vi "XLP80.vi"() -> ()   [LabVIEW 2021]
uses:
  XLP80_General_Libs/WL_Libs_V14.25/WL_TypeDefs_V14.00.llb/WL_TypeDefs_EnumState.ctl
  XLP80_General_Libs/Kirschenhofer_Libs/KH EthernetIPConfig 17.14/KH EthernetIPConfig TDef Config.ctl
  XLP80_General_Libs/Kirschenhofer_Libs/KH EthernetIPConfig 17.14/KH EthernetIPConfig TypeDefs ModuleTyp.ctl
  XLP80_ProjectLibs/XLP80_Globals/XLP80_Globals_SettingsFix.vi
  XLP80_ProjectLibs/XLP80_Globals/XLP80_Globals_Status.vi
  XLP80_General_Libs/WL_Libs_V14.25/WL_Frontpanel_V14.01.llb/WL_Frontpanel_GblStatus.vi
  XLP80_General_Libs/WL_Libs_V14.25/WL_Applications_V14.02.llb/WL_Applications_Globals.vi
  XLP80_General_Libs/Kirschenhofer_Libs/KH EthernetIP 17.19/KH_EthernetIP_Globals.vi
panel:
  out "SW-Version":string
  out "StatusLine":T1={"Status"=1, "code"=0, "source"=""}
  in  "Auto":bool
  in  "EditConf":bool
  in  "Manual":bool
  in  "Info":bool
  in  "Exit":bool
  in  "LoadConf":bool
  # "XLP 80"
  # "XLP 80"
  # "Mess- & Prüfsoftware: m-a-r-s Ing.Büro Wais; www.m-a-r-s.de"
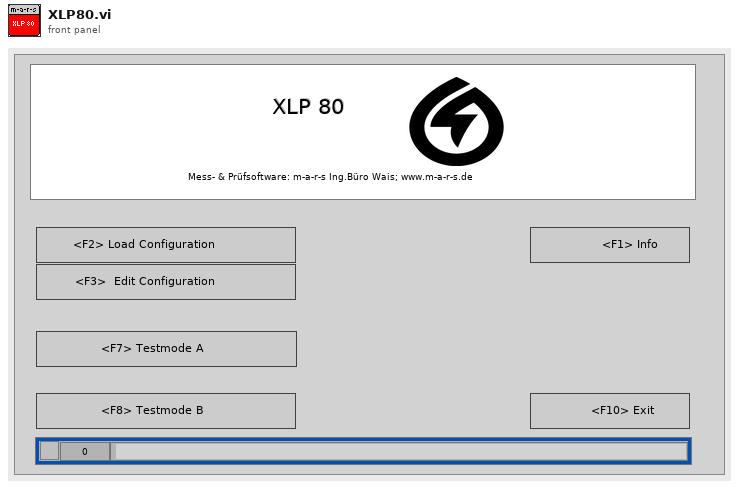
[diagram p1: front panel]
types:
  T1 = cluster{"Status":u16, "code":i32, "source":string}
  T2 = enum32{"General Settings", "Datalog", "Parameter", "AlarmReal", "AlarmBool", "AI", "AO", "DI", "DO", "CAN", "Extra Settings"}
  T3 = typedef "WL_TypeDefs_EnumState.ctl" = enum16{"Init", "Run", "End"}
  T4 = enum16{"-none-", "Info", "LoadConf", "EditConf", "Auto", "Manual", "Exit"}
  T5 = typedef "KH EthernetIPConfig TDef Config.ctl" = cluster{"Typ":T6, "Name":string, "Nr.":i32, "InputOutput":enum16{"Input", "Output"}[]}
  T6 = typedef "KH EthernetIPConfig TypeDefs ModuleTyp.ctl" = enum16{"TBEN-S2-4AI", "TBEN-S1-8DXP", "TBEN-S2-2RFID-4DXP", "TBEN-S2-4AO", "TBEN-S2-4IOL"}
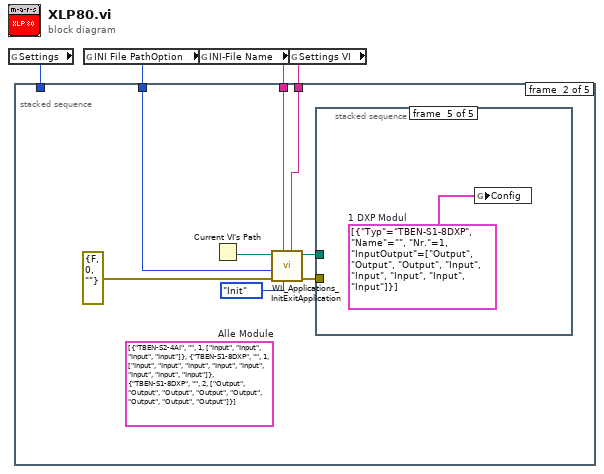
[diagram p0: block diagram]
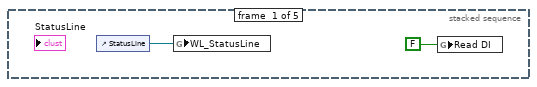
[diagram p2: hidden frame]
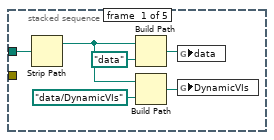
[diagram p3: hidden frame]
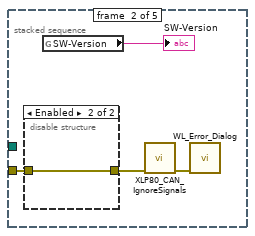
[diagram p4: hidden frame]
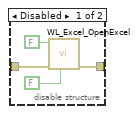
[diagram p5: hidden frame]
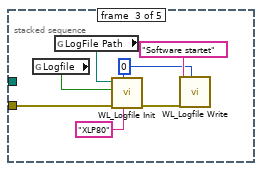
[diagram p6: hidden frame]
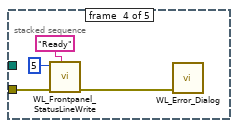
[diagram p7: hidden frame]
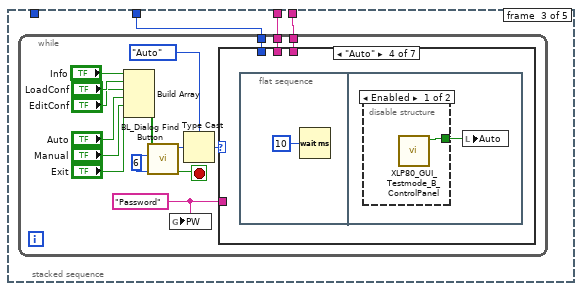
[diagram p8: hidden frame]
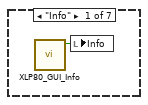
[diagram p9: hidden frame]
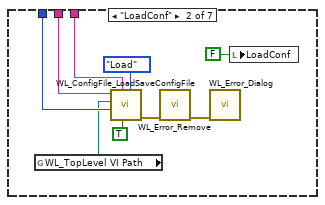
[diagram p10: hidden frame]
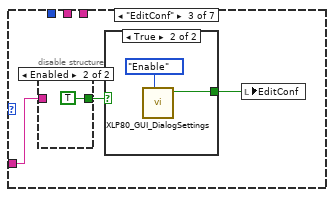
[diagram p11: hidden frame]
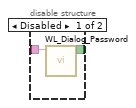
[diagram p12: hidden frame]
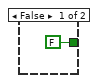
[diagram p13: hidden frame]
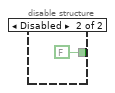
[diagram p14: hidden frame]
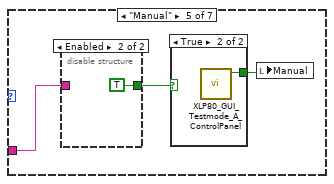
[diagram p15: hidden frame]
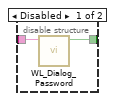
[diagram p16: hidden frame]
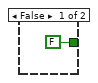
[diagram p17: hidden frame]
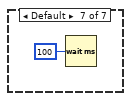
[diagram p19: hidden frame]
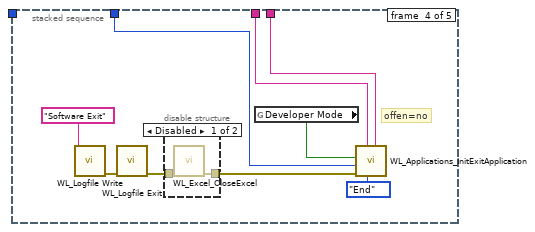
[diagram p20: hidden frame]
diagram:
  n1 = global read "Globals_Settings_XLP80.vi" "Settings"() -> (w1:T2)
  n2 = global read "XLP80_Globals_SettingsFix.vi" "INI File PathOption"() -> (w4:enum16{"WindowsPath", "LocalPath", "Path"})
  n3 = global read "XLP80_Globals_SettingsFix.vi" "INI-File Name"() -> (w3:string)
  n4 = global read "XLP80_Globals_SettingsFix.vi" "Settings VI"() -> (w2:string)
  n5 = stacked-sequence {
    tunnel: w2 -> [_ w12 w44 w99 _]
    tunnel: w3 -> [_ w13 w43 w98 _]
    tunnel: w4 -> [_ w14 w42 w95 _]
    tunnel: w1 -> [_ _ _ _ _]
    frame #0 {
      n6 = control-ref of="StatusLine"() -> (w6:refnum<vi>)
      n7 = global write "WL_Frontpanel_GblStatus.vi" "WL_StatusLine"(w6) -> ()
      n8 = global write "XLP80_Globals_Status.vi" "Read DI"(FALSE ("Read DI")) -> ()
    }
    frame #1 {
      (unwired) T5[] [{"Typ"=enum."TBEN-S2-4AI", "Name"="", "Nr."=1, "InputOutput"=[enum."Input", enum."Input", enum."Input", enum."Input"]}, {"Typ"=enum."TBEN-S1-8DXP", "Name"="", "Nr."=1, "InputOutput"=[enum."Input", enum."Input", enum."Input", enum."Input", enum."Input", enum."Input", enum."Input", enum."Input"]}, {"Typ"=enum."TBEN-S1-8DXP", "Name"="", "Nr."=2, "InputOutput"=[enum."Output", enum."Output", enum."Output", enum."Output", enum."Output", enum."Output", enum."Output", enum."Output"]}]  # Alle Module
      n9 = Current VI's Path() -> (path=w9:path)
      n10 = call "WL_Applications_InitExitApplication.vi"("Settings VI"=w12, "State"=WL_TypeDefs_EnumState."Init", "INI-File Name"=w13, "error in"=errorcluster {"status"=FALSE, "code"=0, "source"=""}, "PathOption"=w14, "Top Level VI Path"=w9) -> ("error out"=w11:errorcluster, "ConfigFile"=w7:path)  [unwired: 4 in]
      n11 = stacked-sequence {
        tunnel: w11 -> [_ w24 w35 w38 _]
        tunnel: w7 -> [w18 _ _ _ _]
        frame #0 {
          n12 = Strip Path(path=w18) -> (stripped path=w16:path)  [unwired: 1 out]
          n13 = Build Path(base path=w16, name or relative path=path "data") -> (appended path=w19:path)
          n14 = Build Path(base path=w16, name or relative path=path "data/DynamicVIs") -> (appended path=w15:path)
          n15 = global write "XLP80_Globals_Status.vi" "data"(w19) -> ()
          n16 = global write "XLP80_Globals_Status.vi" "DynamicVIs"(w15) -> ()
        }
        frame #1 {
          n17 = disable-structure shown="Enabled" {
            disable-tunnel: w24 -> [w28 w29]
            disable-tunnel: [w27 w29] -> w23
            frame Disabled {
              n18 = call "WL_Excel_OpenExcel.vi"("ProgressBar"=FALSE, "error in"=w28, "Visible"=FALSE) -> ("error out"=w27:errorcluster)  [unwired: 6 in, 2 out]
            }
            frame Enabled {
            }
          }
          n19 = global read "WL_Applications_Globals.vi" "SW-Version"() -> (→"SW-Version":string)
          n20 = call "XLP80_CAN_IgnoreSignals.vi"("err in"=w23) -> ("err out"=w22:errorcluster)  [unwired: 10 in]
          n21 = call "WL_Error_Dialog.vi"("err in"=w22) -> ()  [unwired: 10 in, 1 out]
        }
        frame #2 {
          w32 = 0 ("LogfileIndex (0)")
          n22 = global read "Globals_Settings_XLP80.vi" "Logfile"() -> (w30:bool)
          n23 = global read "Globals_Settings_XLP80.vi" "LogFile Path"() -> (w31:path)
          n24 = call "WL_Logfile Init.vi"("GroupName"="XLP80", "LogfileIndex (0)"=w32, "err in"=w35, "Logfile"=w30, "Logfile Path"=w31) -> ("err out"=w33:errorcluster)  [unwired: 5 in, 1 out]
          n25 = call "WL_Logfile Write.vi"("LogfileIndex (0)"=w32, "err in"=w33, "String To LOGfile"="Software startet") -> ()  [unwired: 8 in, 1 out]
        }
        frame #3 {
          n26 = call "WL_Frontpanel_StatusLineWrite.vi"("Message"="Ready", "err in"=w38, "TestStatus"=u16 5) -> ("err out"=w37:errorcluster)  [unwired: 8 in]
          n27 = call "WL_Error_Dialog.vi"("err in"=w37) -> ()  [unwired: 10 in, 1 out]
        }
        frame #4 {
          w41 = T5[] [{"Typ"=enum."TBEN-S1-8DXP", "Name"="", "Nr."=1, "InputOutput"=[enum."Output", enum."Output", enum."Output", enum."Input", enum."Input", enum."Input", enum."Input", enum."Input"]}]  # 1 DXP Modul
          n28 = global write "KH_EthernetIP_Globals.vi" "Config"(w41) -> ()
        }
      }
    }
    frame #2 {
      n29 = while {
        tunnel: w44 -> [w51]
        tunnel: w43 -> [w50]
        tunnel: w42 -> [w48]
        stop <- w54 stop-if-true
        w45 = "Password" ("PW")
        w53 = u16 6 ("first (1..)")
        n30 = Build Array("Info", "LoadConf", "EditConf", "Auto", "Manual", "Exit") -> (w60:bool[])
        n31 = call "BL_Dialog Find Button.vi"("last (1..)"=w53, "first (1..)"=w53, "Buttons"=w60) -> ("Button found"=w54:bool, "U16Button (1...)"=w57:u16)  [unwired: 4 in]
        n32 = global write "XLP80_Globals_Status.vi" "PW"(w45) -> ()
        n33 = Type Cast(type=T4."Auto", x=w57) -> (*(type *) &x=w55:T4)
        n34 = case shown="\"Auto\"" w55 {
          tunnel: w51 -> [_ w70 _ _ _ _ _]
          tunnel: w50 -> [_ w69 _ _ _ _ _]
          tunnel: w48 -> [_ w68 _ _ _ _ _]
          tunnel: w45 -> [_ _ w72 _ w85 _ _]
          frame "Info" {
            n35 = call "XLP80_GUI_Info.vi"() -> ("Boolean"=w61:bool)  [unwired: 6 in, 1 out]
            n36 = local write "Info"(w61) -> ()
          }
          frame "LoadConf" {
            n37 = global read "WL_Frontpanel_GblStatus.vi" "WL_TopLevel VI Path"() -> (w65:path)
            n38 = call "WL_ConfigFile_LoadSaveConfigFile.vi"("Function (Load)"=enum16{"Load", "Save"}."Load", "File Selection? (F)"=TRUE, "Settings Global VI Name"=w70, "PathOption"=w68, "Basepath (CurrentVI if Local)"=w65, "INI-File Name"=w69) -> ("err out"=w64:errorcluster)  [unwired: 4 in, 1 out]
            n39 = call "WL_Error_Remove.vi"("err in"=w64) -> ("err out"=w63:errorcluster)  [unwired: 6 in, 1 out]
            n40 = call "WL_Error_Dialog.vi"("err in"=w63) -> ()  [unwired: 10 in, 1 out]
            n41 = local write "LoadConf"(FALSE ("LoadConf")) -> ()
          }
          frame "EditConf" {
            n42 = disable-structure shown="Enabled" {
              disable-tunnel: w72 -> [w75 _]
              disable-tunnel: [w74 TRUE ("Passed")] -> w71
              frame Disabled {
                n43 = call "WL_Dialog_Password.vi"("PW"=w75) -> ("Passed"=w74:bool)  [unwired: 7 in, 1 out]
              }
              frame Enabled {
              }
            }
            n44 = case shown="True" w71 {
              tunnel: [FALSE ("active (F)") w79] -> w73
              frame False {
              }
              frame True {
                n45 = call "XLP80_GUI_DialogSettings.vi"("State"=enum16{"Enable", "Disable"}."Enable") -> ("active (F)"=w79:bool)  [unwired: 9 in, 1 out]
              }
            }
            n46 = local write "EditConf"(w73) -> ()
          }
          frame "Auto" {
            n47 = flat-sequence {
              frame #0 {
                n48 = Wait (ms)(milliseconds to wait=u32 10) -> ()  [unwired: 1 out]
              }
              frame #1 {
                n49 = disable-structure shown="Enabled" {
                  disable-tunnel: [w82 FALSE ("Auto")] -> w81
                  frame Enabled {
                    n50 = call "XLP80_GUI_Testmode_B_ControlPanel.vi"() -> ("Button (F)"=w82:bool)  [unwired: 10 in, 1 out]
                  }
                  frame Disabled {
                  }
                }
                n51 = local write "Auto"(w81) -> ()
              }
            }
          }
          frame "Manual" {
            n52 = disable-structure shown="Enabled" {
              disable-tunnel: w85 -> [w88 _]
              disable-tunnel: [w87 TRUE ("Passed")] -> w84
              frame Disabled {
                n53 = call "WL_Dialog_Password.vi"("PW"=w88) -> ("Passed"=w87:bool)  [unwired: 7 in, 1 out]
              }
              frame Enabled {
              }
            }
            n54 = case shown="True" w84 {
              tunnel: [FALSE ("Button (F)") w91] -> w86
              frame False {
              }
              frame True {
                n55 = call "XLP80_GUI_Testmode_A_ControlPanel.vi"() -> ("Button (F)"=w91:bool)  [unwired: 10 in, 1 out]
              }
            }
            n56 = local write "Manual"(w86) -> ()
          }
          frame "Exit" {
          }
          frame Default {
            n57 = Wait (ms)(milliseconds to wait=u32 100) -> ()  [unwired: 1 out]
          }
        }
      }
    }
    frame #3 {
      # "offen=no"
      n58 = call "WL_Logfile Write.vi"("String To LOGfile"="Software Exit") -> ("err out"=w100:errorcluster)  [unwired: 10 in]
      n59 = call "WL_Logfile Exit.vi"("err in"=w100) -> ("err out"=w94:errorcluster)  [unwired: 7 in]
      n60 = disable-structure shown="Disabled" {
        disable-tunnel: w94 -> [w103 w104]
        disable-tunnel: [w102 w104] -> w93
        frame Disabled {
          n61 = call "WL_Excel_CloseExcel.vi"("error in"=w103) -> ("error out"=w102:errorcluster)  [unwired: 10 in]
        }
        frame Enabled {
        }
      }
      n62 = global read "Globals_Settings_XLP80.vi" "Developer Mode"() -> (w97:bool)
      n63 = call "WL_Applications_InitExitApplication.vi"("Settings VI"=w99, "State"=WL_TypeDefs_EnumState."End", "INI-File Name"=w98, "error in"=w93, "PathOption"=w95, "Developper Mode"=w97) -> ()  [unwired: 4 in, 2 out]
    }
    frame #4 {
      n64 = local write "Exit"(FALSE ("FileConv")) -> ()
    }
  }
